vi "VI Tree - Large File__ogtk.vi"   [LabVIEW 2017]
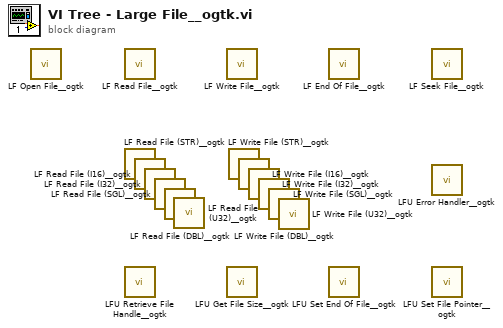
[diagram p0: block diagram]
diagram:
  n1 = call <userlib>:"LF Open File__ogtk.vi"() -> ()  [unwired: 6 in, 2 out]
  n2 = call-poly <userlib>:"LF Read File__ogtk.vi"() -> ()  [unwired: 8 in, 4 out]
  n3 = call <userlib>:"LF Read File (STR)__ogtk.vi"() -> ()  [unwired: 8 in, 4 out]
  n4 = call <userlib>:"LFU Retrieve File Handle__ogtk.vi"() -> ()  [unwired: 6 in, 2 out]
  n5 = call <userlib>:"LF Read File (I16)__ogtk.vi"() -> ()  [unwired: 8 in, 4 out]
  n6 = call <userlib>:"LF Read File (I32)__ogtk.vi"() -> ()  [unwired: 8 in, 4 out]
  n7 = call <userlib>:"LF Read File (SGL)__ogtk.vi"() -> ()  [unwired: 8 in, 4 out]
  n8 = call <userlib>:"LF Read File (DBL)__ogtk.vi"() -> ()  [unwired: 8 in, 4 out]
  n9 = call <userlib>:"LF Read File (U32)__ogtk.vi"() -> ()  [unwired: 8 in, 4 out]
  n10 = call-poly <userlib>:"LF Write File__ogtk.vi"() -> ()  [unwired: 8 in, 3 out]
  n11 = call <userlib>:"LFU Get File Size__ogtk.vi"() -> ()  [unwired: 5 in, 3 out]
  n12 = call <userlib>:"LF Write File (STR)__ogtk.vi"() -> ()  [unwired: 8 in, 3 out]
  n13 = call <userlib>:"LF Write File (I16)__ogtk.vi"() -> ()  [unwired: 8 in, 3 out]
  n14 = call <userlib>:"LF Write File (I32)__ogtk.vi"() -> ()  [unwired: 8 in, 3 out]
  n15 = call <userlib>:"LF Write File (SGL)__ogtk.vi"() -> ()  [unwired: 8 in, 3 out]
  n16 = call <userlib>:"LF Write File (DBL)__ogtk.vi"() -> ()  [unwired: 8 in, 3 out]
  n17 = call <userlib>:"LF Write File (U32)__ogtk.vi"() -> ()  [unwired: 8 in, 3 out]
  n18 = call <userlib>:"LF End Of File__ogtk.vi"() -> ()  [unwired: 5 in, 3 out]
  n19 = call <userlib>:"LFU Set End Of File__ogtk.vi"() -> ()  [unwired: 6 in, 2 out]
  n20 = call <userlib>:"LF Seek File__ogtk.vi"() -> ()  [unwired: 5 in, 3 out]
  n21 = call <userlib>:"LFU Error Handler__ogtk.vi"() -> ()  [unwired: 2 in, 1 out]
  n22 = call <userlib>:"LFU Set File Pointer__ogtk.vi"() -> ()  [unwired: 5 in, 3 out]
